vi "Untitled 2.vi"() -> ()   [LabVIEW 2020]
panel:
  in  "Numeric 5":dbl
  out "Numeric 4":i32
  in  "stop 2":bool
  in  "millisecond timer value 2":u32
  in  "Slide 2":dbl(slide) scale=-50.0..300.0
  out "Thermometer 2":dbl(slide) scale=-100.0..100.0
  out "Numeric 3":dbl
  in  "Boolean 2":bool
  in  "Boolean":bool
  out "Numeric 2":dbl
  out "Thermometer":dbl(slide) scale=-100.0..100.0
  in  "Slide":dbl(slide) scale=-50.0..300.0
  in  "millisecond timer value":u32
  in  "stop":bool
  out "Numeric":i32
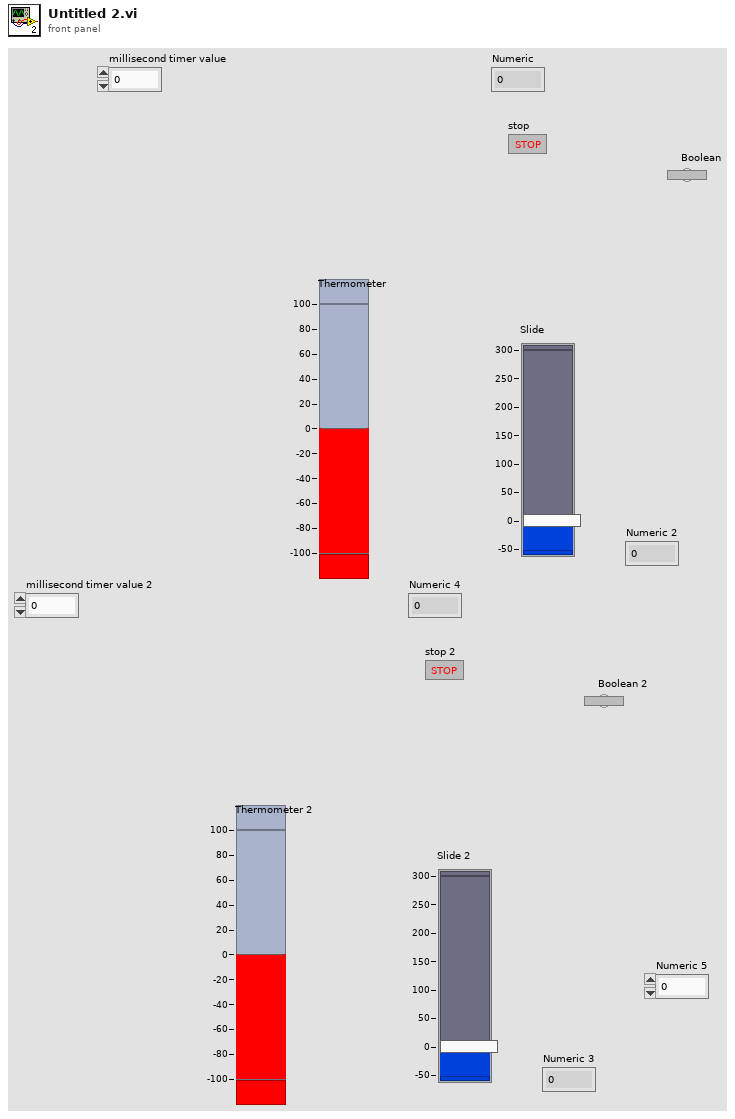
[diagram p1: front panel]
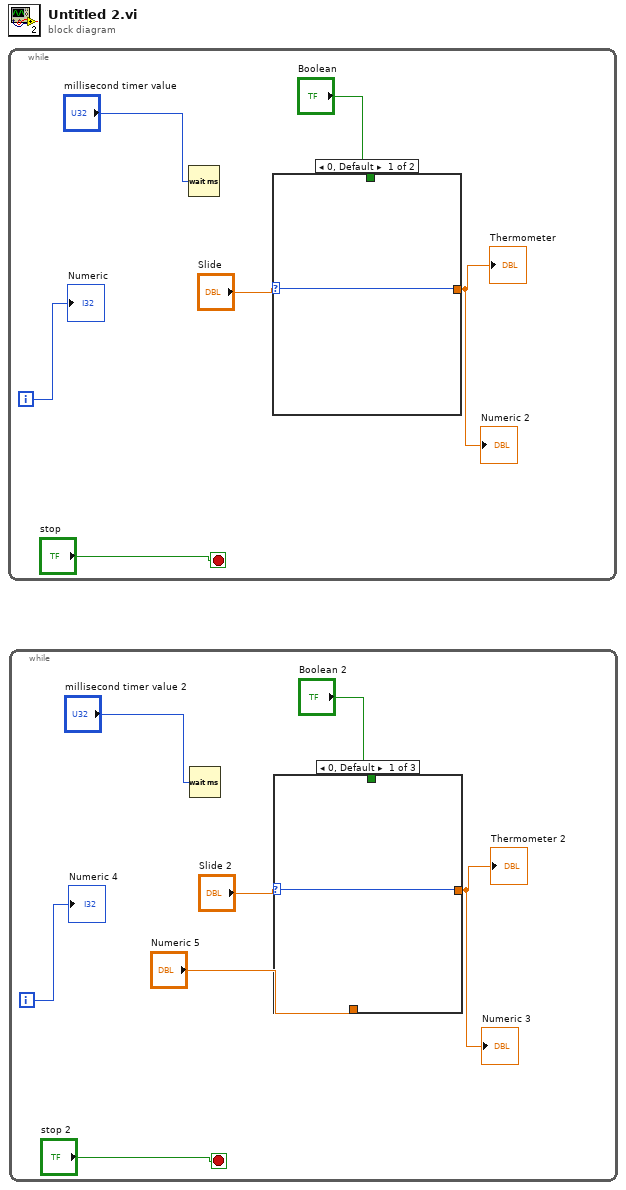
[diagram p0: block diagram]
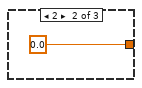
[diagram p2: hidden frame]
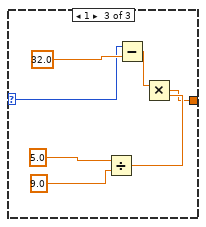
[diagram p3: hidden frame]
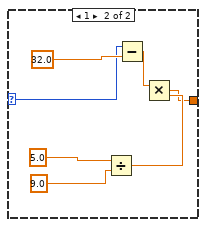
[diagram p4: hidden frame]
diagram:
  n1 = while {
    i -> [w6]
    stop <- "stop" stop-if-true
    n2 = Wait (ms)(milliseconds to wait="millisecond timer value") -> ()  [unwired: 1 out]
    n3 = case shown="0, Default" "Slide" {
      selector: "Slide" -> [w7 w8]
      tunnel: [w7 w10] -> w3
      tunnel: "Boolean" -> [_ _]
      frame 0, Default {
      }
      frame 1 {
        n4 = Divide(x=5.0, y=9.0 ("x")) -> (x/y=w11:dbl)
        n5 = Subtract(x=w8, y=32.0) -> (x-y=w12:dbl)
        n6 = Multiply(x=w12, y=w11) -> (x*y=w10:dbl)
      }
    }
    "Thermometer" <- w3
    "Numeric 2" <- w3
    "Numeric" <- w6
  }
  n7 = while {
    i -> [w21]
    stop <- "stop 2" stop-if-true
    n8 = Wait (ms)(milliseconds to wait="millisecond timer value 2") -> ()  [unwired: 1 out]
    n9 = case shown="0, Default" "Slide 2" {
      selector: "Slide 2" -> [w22 _ w24]
      tunnel: [w22 0.0 ("Numeric 5") w26] -> w18
      tunnel: "Boolean 2" -> [_ _ _]
      tunnel: "Numeric 5" -> [_ _ _]
      frame 0, Default {
      }
      frame 2 {
      }
      frame 1 {
        n10 = Divide(x=5.0, y=9.0 ("x")) -> (x/y=w27:dbl)
        n11 = Subtract(x=w24, y=32.0) -> (x-y=w28:dbl)
        n12 = Multiply(x=w28, y=w27) -> (x*y=w26:dbl)
      }
    }
    "Thermometer 2" <- w18
    "Numeric 3" <- w18
    "Numeric 4" <- w21
  }
